vi "Is Empty.vi"(3 "IMsgPackContainer in":refnum<class "IMsgPackContainer.lvclass">) -> (1 "Is empty?":bool=TRUE)   [LabVIEW 2020, in "MessagePack.lvlib" / "IMsgPackContainer.lvclass"]
uses:
  IMsgPackContainer.lvclass
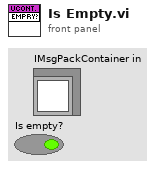
[diagram p1: front panel]
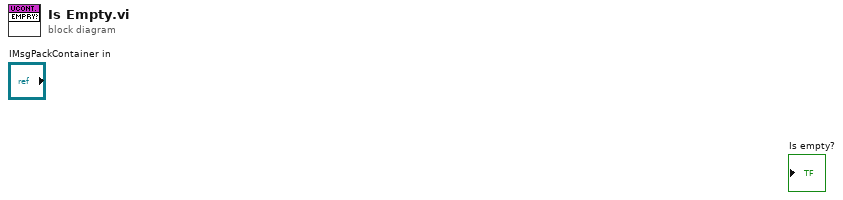
[diagram p0: block diagram]
diagram:
